vi "util_stddev_variance.vi"(0 "X":dbl[](array[numeric]) format="%0.2f", 1 "Weighting (Sample)":enum16{"Sample", "Population"}(ring)) -> (2 "mean":dbl format="%0.2f", 3 "standard deviation":dbl format="%0.2f", 4 "variance":dbl format="%0.2f")   [LabVIEW 2016]
doc: "Computes the mean, std. deviation snd variance of the input array. The latter two default to 0 when array has length 0 or 1."
uses:
  <vilib>/Analysis/NI_AALBase.lvlib
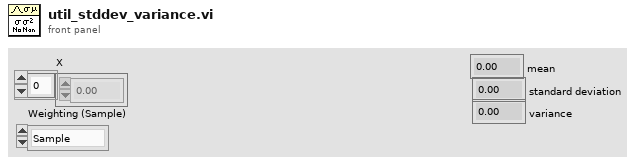
[diagram p1: front panel]
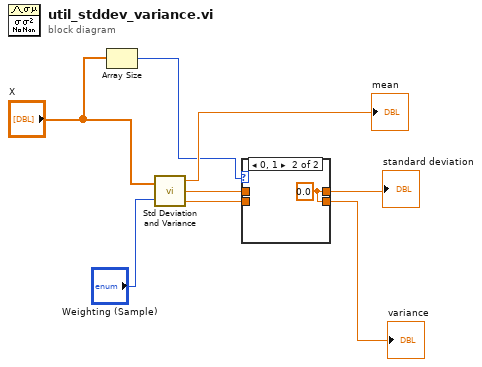
[diagram p0: block diagram]
diagram:
  n1 = Array Size(array="X") -> (size(s)=w5:i32)
  n2 = call <vilib>:"Std Deviation and Variance.vi"("X"="X", "Weighting (Sample)"="Weighting (Sample)") -> ("mean"=→"mean":dbl, "standard deviation"=w4:dbl, "variance"=w3:dbl)
  n3 = case shown="0, 1" w5 {
    tunnel: w4 -> [w9 _]
    tunnel: w3 -> [w10 _]
    tunnel: [w10 w11] -> w2
    tunnel: [w9 w11] -> w1
    frame Default {
    }
    frame 0, 1 {
      w11 = 0.0 ("standard deviation")
    }
  }
  "standard deviation" <- w1
  "variance" <- w2
